vi "Checkers New Game.vi"   [LabVIEW 2016]
panel:
  # "If you're reading this, \nthis VI isn't doing it's job correctly."
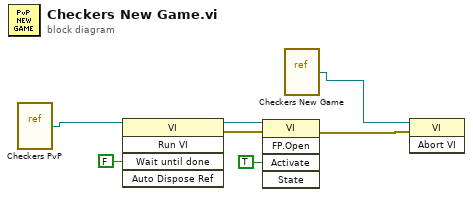
[diagram p0: block diagram]
diagram:
  n1 = vi-ref "Checkers PvP.vi"() -> (w7:refnum<vi>)
  n2 = invoke class="VI" method="Run VI"(reference=w7, "Wait until done"=FALSE ("Wait Until Done")) -> (reference out=w6:refnum<vi>, error out=w5:errorcluster)  [unwired: 3 in, 3 out]
  n3 = invoke class="VI" method="FP.Open"(reference=w6, error in=w5, "Activate"=TRUE ("Activate?")) -> (error out=w4:errorcluster)  [unwired: 2 in, 4 out]
  n4 = vi-ref "Checkers New Game.vi"() -> (w1:refnum<vi>)
  n5 = invoke class="VI" method="Abort VI"(reference=w1, error in=w4) -> ()  [unwired: 1 in, 3 out]
